vi "mclb_font.vi"(8 "error in (no error)":errorcluster, 11 "mclb in":refnum<vi>) -> (0 "error out":errorcluster, 2 "default font":T1, 3 "mclb out":refnum<vi>)   [LabVIEW 2017, in "rywindow.lvclass"]
uses:
  rywindow.lvclass
  <vilib>/Utility/miscctls.llb/LVFontTypeDef.ctl
  <vilib>/Utility/miscctls.llb/LVRowAndColumnUnsignedTypeDef.ctl
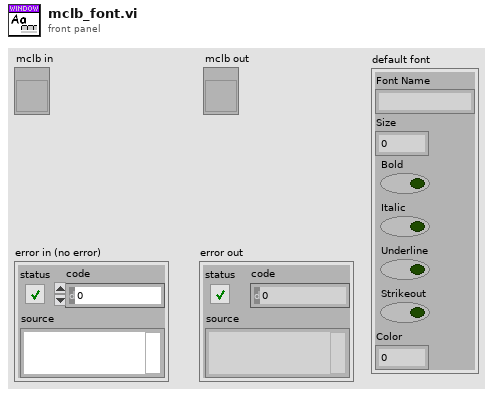
[diagram p1: front panel]
types:
  T1 = typedef "LVFontTypeDef.ctl" = cluster{"Font Name":string, "Size":u16, "Bold":bool, "Italic":bool, "Underline":bool, "Strikeout":bool, "Color":u32}
  T2 = typedef "LVRowAndColumnUnsignedTypeDef.ctl" = cluster{"Row":u32, "Column":u32}
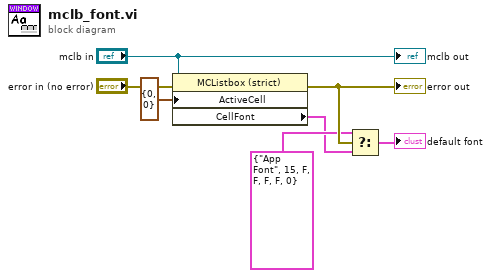
[diagram p0: block diagram]
diagram:
  n1 = property class="MCListbox (strict)"(reference="mclb in", error in="error in (no error)", "ActiveCell"=T2 {"Row"=0, "Column"=0} ("Top Left Visible Cell")) -> (error out=w5:errorcluster, "CellFont"=w3:T1)  [unwired: 1 out]
  "error out" <- w5
  n2 = Select(t=T1 {"Font Name"="App Font", "Size"=15, "Bold"=FALSE, "Italic"=FALSE, "Underline"=FALSE, "Strikeout"=FALSE, "Color"=0} ("default font"), s=w5, f=w3) -> (s? t:f=→"default font":T1)
  "mclb out" <- "mclb in"
